vi "ScanAction.vi"(8 "error in (no error)":errorcluster caption="entrée d'erreur (pas d'erreur)", 9 "IndicePoint":i32, 11 "Spex In":refnum<class "Spex.lvclass"> caption="DNL_LabVIEW Object in") -> (0 "error out":errorcluster caption="sortie d'erreur", 2 "ScanParsOut":dbl[](array[numeric]), 3 "Spex Out":refnum<class "Spex.lvclass"> caption="DNL_LabVIEW Object out")   [LabVIEW 2019, in "Spex.lvclass"]
uses:
  Spex.lvclass
  C:/Programmes Labview/LabScanV1A/DevicesClass/BaseDevice/BaseDevice.lvclass
  Spex.lvclass/Spex.ctl
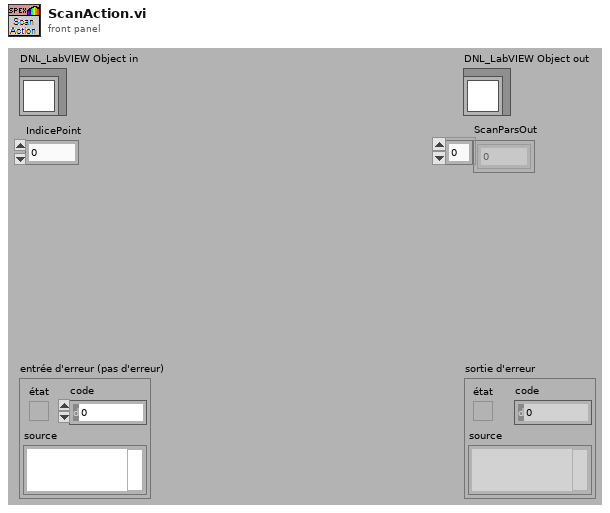
[diagram p1: front panel]
types:
  T1 = typedef "Spex.lvclass/Spex_Func.ctl" = enum16{"Position (nm)"}
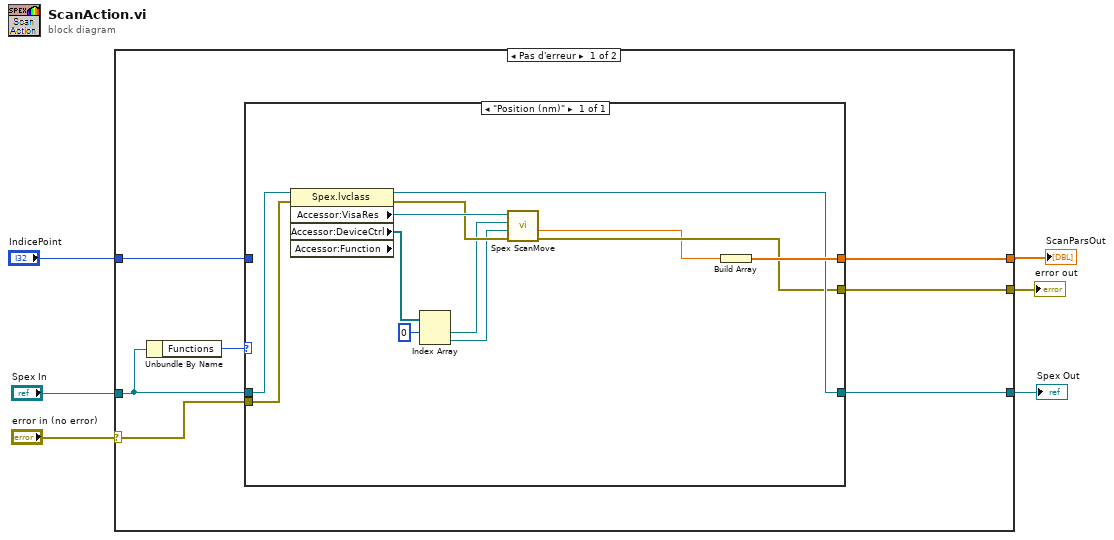
[diagram p0: block diagram]
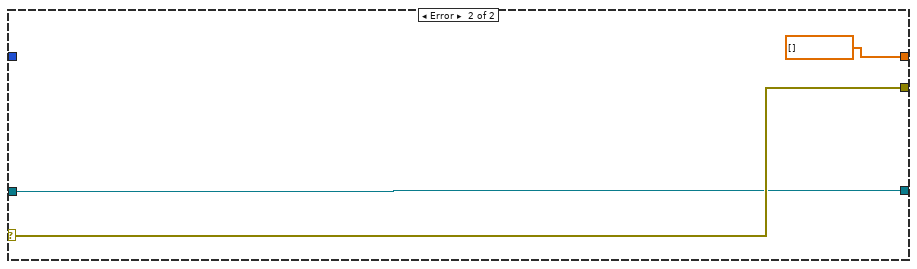
[diagram p2: hidden frame]
diagram:
  n1 = case shown="Pas d'erreur" "error in (no error)" {
    selector: "error in (no error)" -> [w10 w28]
    tunnel: "Spex In" -> [w11 w27]
    tunnel: [w9 dbl[] []] -> w1
    tunnel: [w8 w28] -> w4
    tunnel: [w7 w27] -> w3
    tunnel: "IndicePoint" -> [w12 _]
    frame No Error {
      n2 = Unbundle By Name(w11) -> ("Functions"=w13:T1)
      n3 = case shown="\"Position (nm)\"" w13 {
        tunnel: [w25] -> w9
        tunnel: w12 -> [_]
        tunnel: [w23] -> w7
        tunnel: w11 -> [w24]
        tunnel: w10 -> [w22]
        tunnel: [w19] -> w8
        frame "Position (nm)" {
          n4 = property class="Spex.lvclass" props=["Accessor:VisaRes", "Accessor:DeviceCtrl", "Accessor:Function"](reference=w24, error in=w22) -> (reference out=w23:refnum<class "Spex.lvclass">, error out=w20:errorcluster, "Accessor:VisaRes"=w21:refnum<visa-resource-name>, "Accessor:DeviceCtrl"=w18:refnum<vi>[])  [unwired: 1 out]
          n5 = Index Array(array=w18, index #1=0 ("indice")) -> (element #1=w16:refnum<vi>, element #2=w15:refnum<vi>)  [unwired: 1 in]
          n6 = call <userlib>:"Spex ScanMove.vi"("error in"=w20, "Moving Ref"=w15, "Lambda Ref"=w16, "Port"=w21) -> ("error out"=w19:errorcluster, "Wlenght"=w14:dbl)  [unwired: 3 in, 3 out]
          n7 = Build Array(w14) -> (w25:dbl[])
        }
      }
    }
    frame Error {
    }
  }
  "error out" <- w4
  "Spex Out" <- w3
  "ScanParsOut" <- w1
